vi "(SubVI) EQP method_YCC.vi"(3 "Sensitivity (V/um)":dbl, 5 "position (V)":dbl[](array[numeric])) -> (0 "variance (V)":dbl format="%0.2f", 1 "k (pN/nm)":dbl)   [LabVIEW 2014]
uses:
  <vilib>/Analysis/NI_AALBase.lvlib
panel:
  in  "Temp (C)":dbl=24.0
  out "STD (nm)":dbl format="%0.2f"
  out "position (nm)":dbl[](array[numeric])
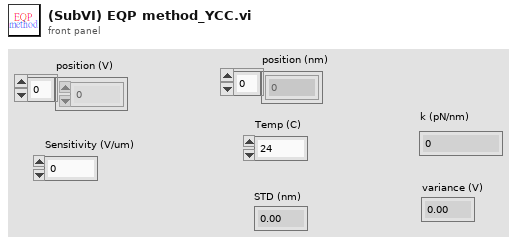
[diagram p1: front panel]
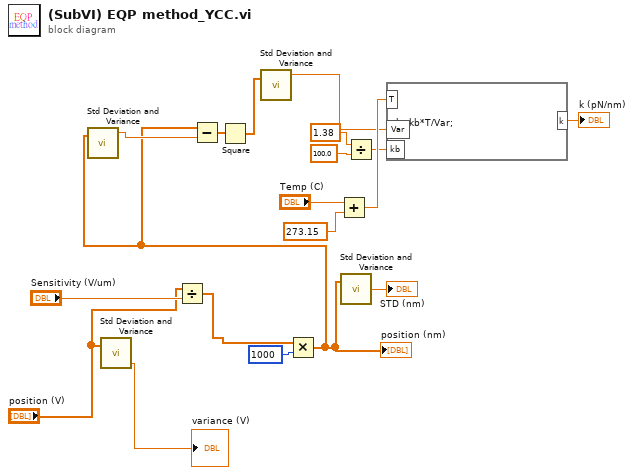
[diagram p0: block diagram]
diagram:
  n1 = call <vilib>:"Std Deviation and Variance.vi"("X"="position (V)") -> ("variance"=→"variance (V)":dbl)  [unwired: 1 in, 2 out]
  n2 = Divide(x="position (V)", y="Sensitivity (V/um)") -> (x/y=w7:dbl[])
  n3 = Multiply(x=w7, y=1000) -> (x*y=w4:dbl[])
  "position (nm)" <- w4
  n4 = call <vilib>:"Std Deviation and Variance.vi"("X"=w4) -> ("mean"=w5:dbl)  [unwired: 1 in, 2 out]
  n5 = Subtract(x=w4, y=w5) -> (x-y=w3:dbl[])
  n6 = Square(x=w3) -> (x^2=w2:dbl[])
  n7 = call <vilib>:"Std Deviation and Variance.vi"("X"=w2) -> ("mean"=w1:dbl)  [unwired: 1 in, 2 out]
  n8 = Add(x="Temp (C)", y=273.15) -> (x+y=w14:dbl)
  n9 = call <vilib>:"Std Deviation and Variance.vi"("X"=w4) -> ("standard deviation"=→"STD (nm)":dbl)  [unwired: 1 in, 2 out]
  n10 = Divide(x=1.38 ("input variable"), y=100.0) -> (x/y=w10:dbl)
  n11 = formula code="k=kb*T/Var;"("T"=w14, "Var"=w1, "kb"=w10) -> ("k"=→"k (pN/nm)":dbl)
